vi "Deserialize Data.vi"(8 "error in (no error)":errorcluster, 11 "Flat Data in":string) -> (0 "error out":errorcluster, 3 "Process Data out":T1)   [LabVIEW 2020, in "Ethernet Frame.lvlib"]
doc: "Version 0.1"
uses:
  <vilib>/ADAS Record/CustomDataTypes/Ethernet Frame/Ethernet Frame.lvlib
  <vilib>/ADAS Record/CustomDataTypes/Ethernet Frame/Process Data.ctl
  <vilib>/ADAS Record/IODataPEF/CfgMgr/FlatFormat.ctl
  5e2451cd-7b8c-4079-9add-41a600a01e16.vi
  <vilib>/ADAS Record/IODataPEF/Error/Error_SetError.vi
  <vilib>/ADAS Record/IODataPEF/Error/Error_CheckAndSetDllError.vi
  <vilib>/ADAS Record/IODataPEF/Error/ErrorMgr.vi
  <vilib>/ADAS Record/CustomData/_Custom_RegisterType.vi
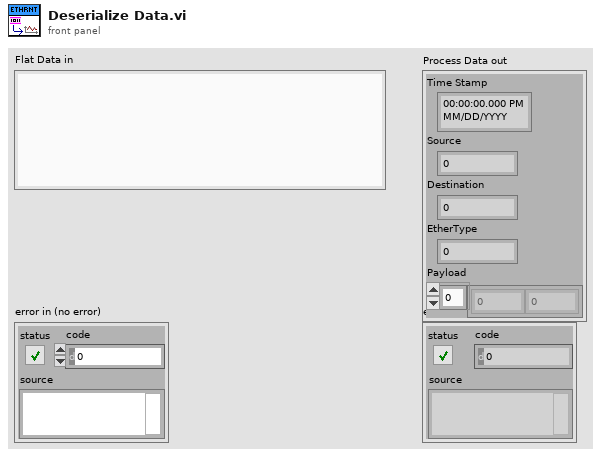
[diagram p1: front panel]
types:
  T1 = typedef "Ethernet Frame.lvlib/Process Data.ctl" = cluster{"Time Stamp":timestamp, "Source":u64, "Destination":u64, "EtherType":u16, "Payload":u8[]}
  T2 = typedef "FlatFormat.ctl" = enum32{"Auto", "PEF", "GFB (Apache)", "GFB", "JSON", "Readable JSON", "LV String", "Reserved", "LV Native"}
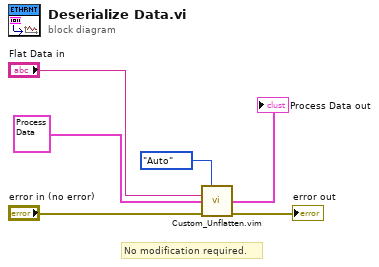
[diagram p0: block diagram]
diagram:
  # "No modification required."
  n1 = call "Custom_Unflatten.vim"("Flat Format"=FlatFormat."Auto", "Flat Data"="Flat Data in", "Data (type/default value)"=T1 {"Time Stamp"=timestamp(0 s since 1904-01-01), "Source"=0, "Destination"=0, "EtherType"=0, "Payload"=[]} ("Byte Array in"), "error in (no error)"="error in (no error)") -> ("Data"=→"Process Data out":T1, "Error (out)"=→"error out":errorcluster)  [unwired: 10 in]
